vi "Handle Errors.vi"(8 "Error In":errorcluster, 9 "LinxStatus":T7, 10 "Function Name":string, 11 "LINX Resource":T1) -> (0 "Error Out":errorcluster, 3 "LINX Resource":T1)   [LabVIEW 2014, in "LMH-LINX.lvlib" / "Local IO.lvlib"]
uses:
  Local IO.lvlib
  Type Defs/LINX Ref.ctl
  Type Defs/Platform.ctl
  Type Defs/Interface.ctl
  Device/Type Defs/LINX Device Config.ctl
  Device/Type Defs/TCP Config.ctl
  Device/Type Defs/Channels.ctl
  Type Defs/LinxStatus.ctl
  Type Defs/Error Type.ctl
  LMH-LINX.lvlib
  Device/Device.lvlib
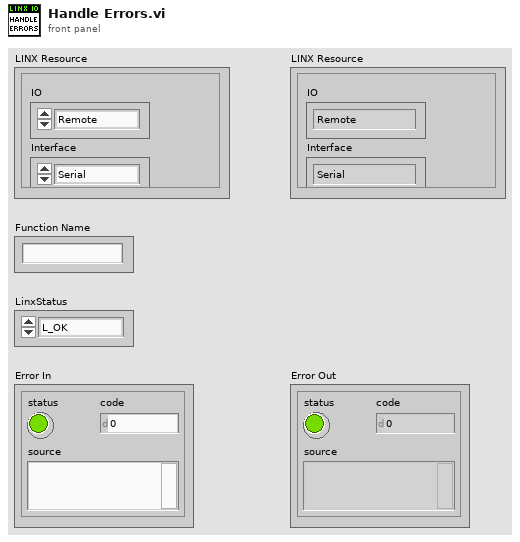
[diagram p1: front panel]
types:
  T1 = typedef "LMH-LINX.lvlib/LINX Ref.ctl" = cluster{"IO":T2, "Interface":T3, "LINX Device Config":T4}
  T2 = typedef "LMH-LINX.lvlib/Platform.ctl" = enum16{"Remote", "Local"}
  T3 = typedef "LMH-LINX.lvlib/Interface.ctl" = enum16{"Serial", "TCP"}
  T4 = typedef "LMH-LINX.lvlib/Device.lvlib/LINX Device Config.ctl" = cluster{"Interface":T3, "COM Port":refnum<visa-resource-name>, "TCP Configuration":T5, "Device Family":u8, "Device ID":u8, "Device Name":string, "TCP Ref":refnum<k5>, "Channels":T6}
  T5 = typedef "LMH-LINX.lvlib/Device.lvlib/TCP Config.ctl" = cluster{"IP Address":string, "Port":u16}
  T6 = typedef "LMH-LINX.lvlib/Channels.ctl" = cluster{"DI":u8[], "DO":u8[], "AI":u8[], "AO":u8[], "PWM":u8[], "QE":u8[], "UART":u8[], "I2C 2":u8[], "SPI":u8[], "CAN":u8[], "Servo":u8[], "AI Ref (V)":dbl, "AO Ref (V)":dbl, "AO Resolution (Bits)":u8}
  T7 = typedef "LMH-LINX.lvlib/Local IO.lvlib/LinxStatus.ctl" = enum32{"L_OK", "L_FUNCTION_NOT__SUPPORTED", "L_REQUEST_RESEND", "L_UNKNOWN_ERROR", "L_DISCONNECT"}
  T8 = typedef "LMH-LINX.lvlib/Error Type.ctl" = enum16{"Unknown", "Timeout", "Corrupt Return Packet", "Unable To Connect", "Command Not Supported", "Channel DNE", "Invalid COM Config", "Firmware Version Mismatch", "myRIO Support", "CMD Specific Error"}
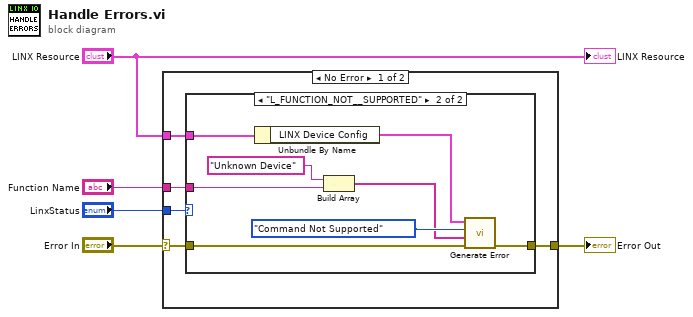
[diagram p0: block diagram]
diagram:
  n1 = case shown="No Error" "Error In" {
    selector: "Error In" -> [w9 w20]
    tunnel: "LinxStatus" -> [w10 _]
    tunnel: [w8 w20] -> w3
    tunnel: "LINX Resource" -> [w7 _]
    tunnel: "Function Name" -> [w6 _]
    frame No Error {
      n2 = case shown="\"L_FUNCTION_NOT__SUPPORTED\"" w10 {
        tunnel: w9 -> [w11 w19]
        tunnel: [w11 w18] -> w8
        tunnel: w7 -> [_ w13]
        tunnel: w6 -> [_ w16]
        frame "L_OK", Default {
        }
        frame "L_FUNCTION_NOT__SUPPORTED" {
          n3 = Unbundle By Name(w13) -> ("LINX Device Config"=w12:T4)
          n4 = Build Array("Unknown Device" ("element"), w16) -> (w15:string[])
          n5 = call "Generate Error.vi"("Error In"=w19, "Arguments"=w15, "Error Type"=Error_Type."Command Not Supported", "LINX Device Config"=w12) -> ("Error Out"=w18:errorcluster)  [unwired: 6 in, 1 out]
        }
      }
    }
    frame Error {
    }
  }
  "Error Out" <- w3
  "LINX Resource" <- "LINX Resource"
